vi "Shutdown.vi"(8 "error in":errorcluster, 11 "nPAS in":refnum<class "nPAS.lvclass">) -> (0 "error out":errorcluster, 3 "nPAS out":refnum<class "nPAS.lvclass">)   [LabVIEW 2017, in "gPAS Library.lvlib" / "nPAS.lvclass"]
doc: "Shutoff the DC power which will control all outputs, close all references to DAQmx tasks and shutoff the laser AO."
uses:
  nPAS.lvclass
  Session/Raw FPGA/FPGA Session.lvclass
  C:/Program Files (x86)/National Instruments/LabVIEW 2017/vi.lib/MSR Consulting, LLC/General Reuse/Session APIs/_Session Fwk/Session - Root.lvclass
  nPAS.lvclass/nPAS.ctl
  <vilib>/MSR Consulting, LLC/General Reuse/PAS/Main/PAS.lvclass
  <vilib>/MSR Consulting, LLC/General Reuse/Session APIs/_Session Fwk/Session - Root.lvclass
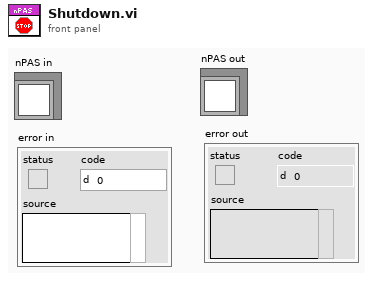
[diagram p1: front panel]
types:
  T1 = typedef "Session - Root.lvclass/Session Handle.ctl" = refnum<data-value>
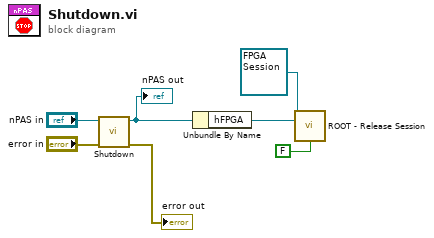
[diagram p0: block diagram]
diagram:
  n1 = call-parent "Shutdown.vi"("error in"="error in", "Instrument in"="nPAS in") -> ("error out"=→"error out":errorcluster, "Instrument out"=w4:refnum<class "nPAS.lvclass">)  [unwired: 8 in]
  "nPAS out" <- w4
  n2 = Unbundle By Name(w4) -> ("hFPGA"=w3:T1)
  n3 = call <vilib>:"ROOT - Release Session.vi"("OBJ - Session in"=refnum<class "FPGA Session.lvclass"> refnum ("FPGA Session"), "Session Handle in"=w3, "force destroy? (F)"=FALSE) -> ()  [unwired: 11 in, 2 out]
